vi "Get Single Tag Value.vi"(8 "Error In":errorcluster, 10 "Tag Name":string, 11 "Element In":refnum<k20>) -> (0 "Error Out":errorcluster, 1 "Tag Value":string, 2 "Tag Reference":refnum<k20>, 3 "Element Out":refnum<k20>)   [LabVIEW 2016, in "Tree Manager.lvclass"]
doc: "From the children of the wired element select only one child node with a matching name. Errors are returned if there is zero or more than one node with this name."
uses:
  Tree Manager.lvclass
  <resource>/objmgr/DOMUserDefRef.rc
  <vilib>/xml/NI_XML.lvlib
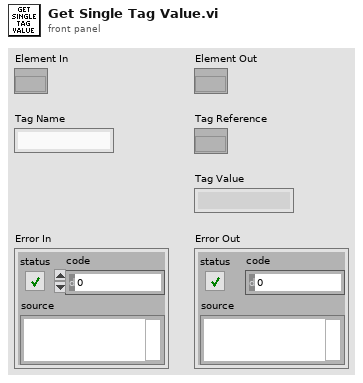
[diagram p1: front panel]
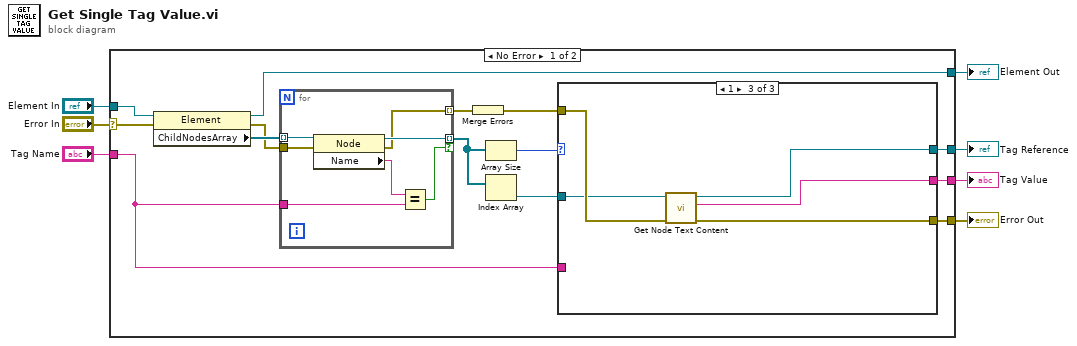
[diagram p0: block diagram]
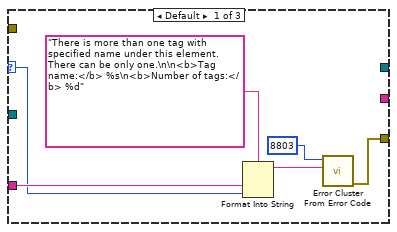
[diagram p2: hidden frame]
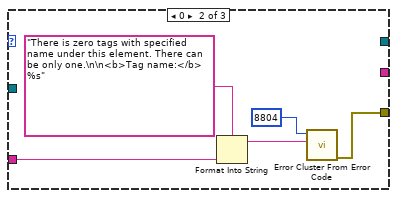
[diagram p3: hidden frame]
diagram:
  n1 = case shown="No Error" "Error In" {
    selector: "Error In" -> [w12 w45]
    tunnel: [w21 _] -> w7
    tunnel: "Tag Name" -> [w14 _]
    tunnel: [w10 w46] -> w5
    tunnel: "Element In" -> [w16 w46]
    tunnel: [w20 w45] -> w3
    tunnel: [w18 _] -> w1
    frame No Error {
      n2 = property class="Element"(reference=w16, error in=w12) -> (reference out=w10:refnum<k20>, error out=w13:errorcluster, "ChildNodesArray"=w15:refnum<k20>[])
      n3 = for {
        tunnel: w15 -> [w28] mode=indexing
        tunnel: w14 -> [w26]
        tunnel: [w25] -> w11 mode=indexing if=w24
        tunnel: w13 -> [w23]
        tunnel: [w22] -> w9 mode=indexing
        n4 = property class="Node"(reference=w28, error in=w23) -> (reference out=w25:refnum<k20>, error out=w22:errorcluster, "Name"=w27:string)
        n5 = Equal?(x=w27, y=w26) -> (x = y?=w24:bool)
      }
      n6 = Merge Errors(w9) -> (w8:errorcluster)
      n7 = Array Size(array=w11) -> (size(s)=w19:i32)
      n8 = Index Array(array=w11) -> (element=w17:refnum<k20>)  [unwired: 1 in]
      n9 = case shown="1" w19 {
        selector: w19 -> [w30 _ _]
        tunnel: [_ _ w44] -> w21
        tunnel: w8 -> [_ _ w43]
        tunnel: w17 -> [_ _ w41]
        tunnel: [w29 w38 w42] -> w20
        tunnel: w14 -> [w31 w39 _]
        tunnel: [_ _ w40] -> w18
        frame Default {
          n10 = Format Into String(format string="There is more than one tag with specified name under this element. There can be only one.\n\n<b>Tag name:</b> %s\n<b>Number of tags:</b> %d", w31, w30) -> (resulting string=w34:string)  [unwired: 2 in, 1 out]
          n11 = call <vilib>:"Error Cluster From Error Code.vi"("error message (\"\")"=w34, "error code (0)"=8803) -> ("error out"=w29:errorcluster)  [unwired: 7 in]
        }
        frame 0 {
          n12 = Format Into String(format string="There is zero tags with specified name under this element. There can be only one.\n\n<b>Tag name:</b> %s", w39) -> (resulting string=w37:string)  [unwired: 2 in, 1 out]
          n13 = call <vilib>:"Error Cluster From Error Code.vi"("error message (\"\")"=w37, "error code (0)"=8804) -> ("error out"=w38:errorcluster)  [unwired: 7 in]
        }
        frame 1 {
          n14 = call <vilib>:"Get Node Text Content.vi"("error in (no error)"=w43, "node in"=w41) -> ("error out"=w42:errorcluster, "node text"=w44:string, "node out"=w40:refnum<k20>)  [unwired: 7 in]
        }
      }
    }
    frame Error {
    }
  }
  "Tag Value" <- w7
  "Error Out" <- w3
  "Element Out" <- w5
  "Tag Reference" <- w1
